vi "Просмотр графиков.vi"() -> ()   [LabVIEW 2011]
panel:
  out "т1 2":waveform(dbl)[](graph)
  out "т1":waveform(dbl)[](graph)
  in  "Закрыть окно":bool
  in  "Сохранить":bool
  # "С1"
  # "С2"
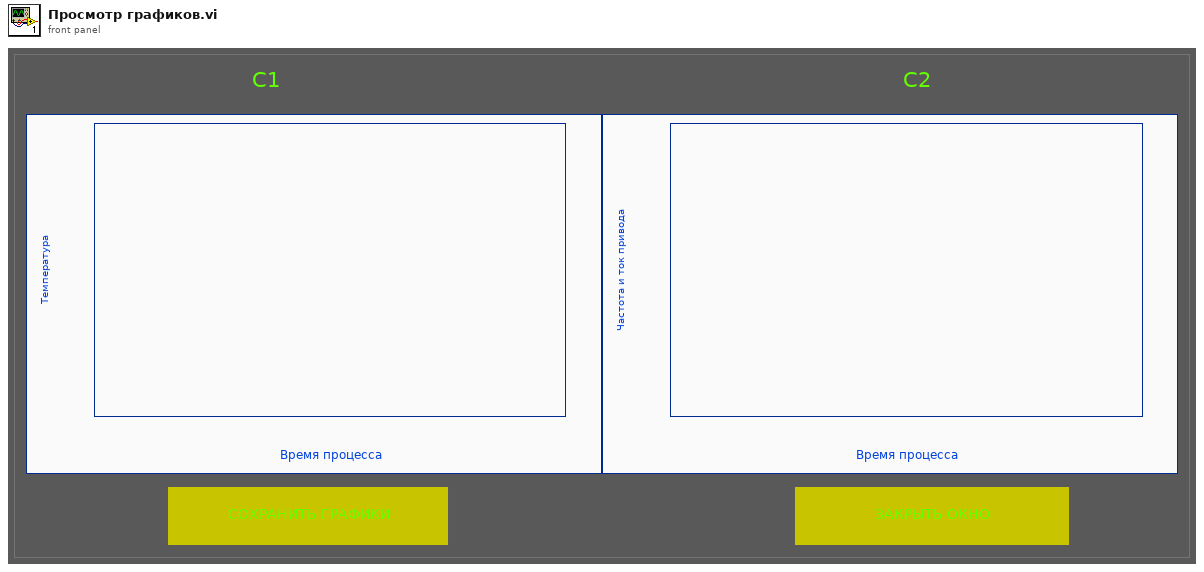
[diagram p1: front panel]
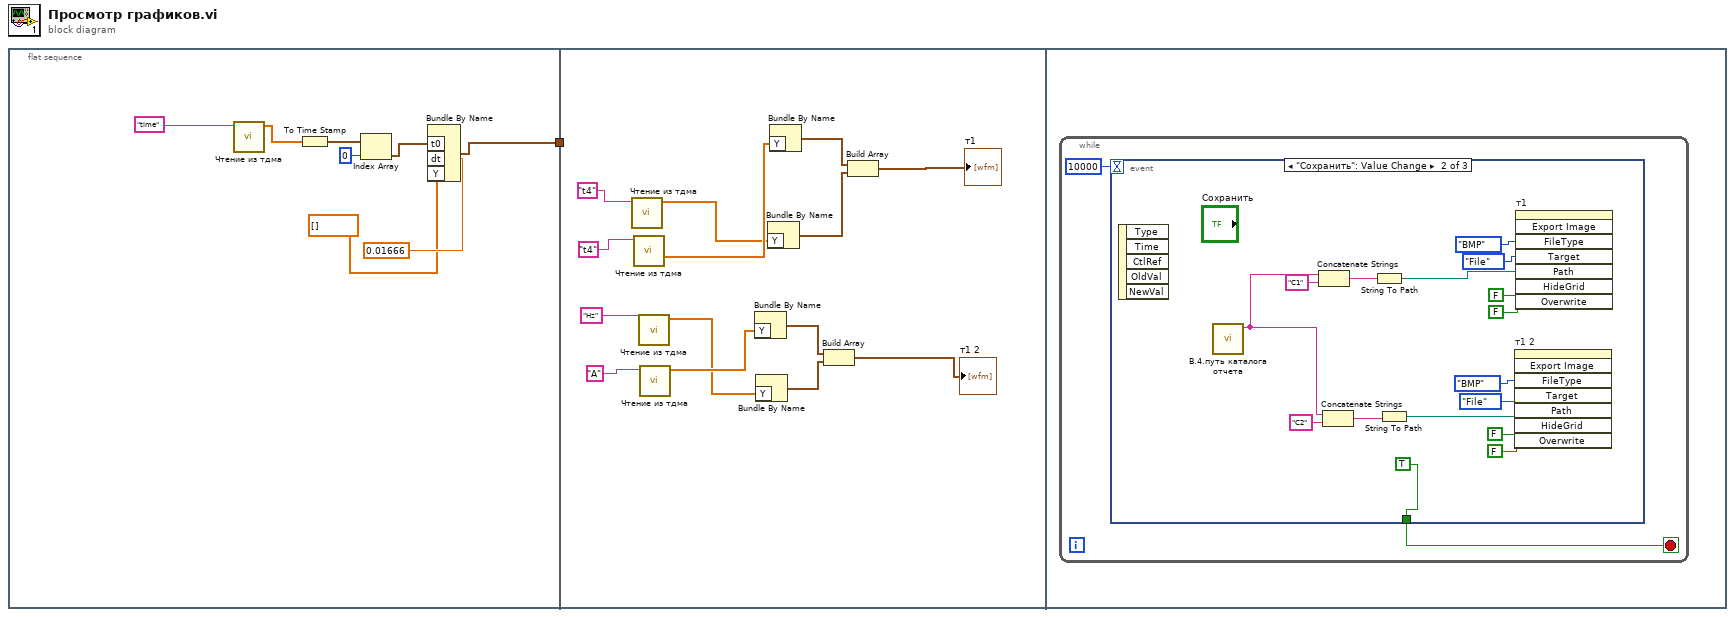
[diagram p0: block diagram]
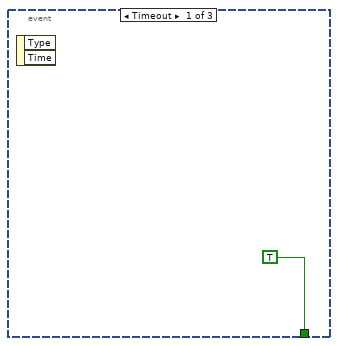
[diagram p2: hidden frame]
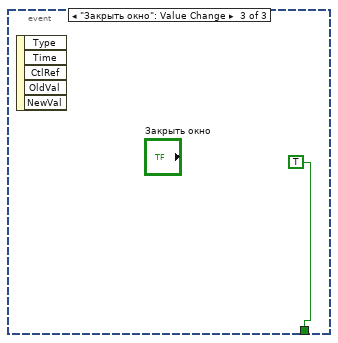
[diagram p3: hidden frame]
diagram:
  n1 = flat-sequence {
    tunnel: [w2] -> w1
    tunnel: w1 -> [_]
    frame #0 {
      n2 = call "Чтение из тдма.vi"("Канал"="time") -> ("data"=w7:dbl[])  [unwired: 10 in]
      n3 = To Time Stamp(1:w7) -> (0:w6:timestamp[])
      n4 = Index Array(array=w6, index=0) -> (element=w3:timestamp)
      n5 = Bundle By Name("t0"=w3, "dt"=0.01666, "Y"=dbl[] []) -> (w2:waveform(dbl))  [unwired: 1 in]
    }
    frame #1 {
      n6 = call "Чтение из тдма.vi"("Канал"="t4") -> ("data"=w10:dbl[])  [unwired: 10 in]
      n7 = call "Чтение из тдма.vi"("Канал"="t4") -> ("data"=w11:dbl[])  [unwired: 10 in]
      n8 = call "Чтение из тдма.vi"("Канал"="Hz") -> ("data"=w12:dbl[])  [unwired: 10 in]
      n9 = call "Чтение из тдма.vi"("Канал"="A") -> ("data"=w13:dbl[])  [unwired: 10 in]
      n10 = Bundle By Name("Y"=w13) -> (w15:waveform(dbl))  [unwired: 1 in]
      n11 = Bundle By Name("Y"=w12) -> (w16:waveform(dbl))  [unwired: 1 in]
      n12 = Bundle By Name("Y"=w10) -> (w20:waveform(dbl))  [unwired: 1 in]
      n13 = Bundle By Name("Y"=w11) -> (w21:waveform(dbl))  [unwired: 1 in]
      n14 = Build Array(w15, w16) -> (→"т1 2":waveform(dbl)[])
      n15 = Build Array(w21, w20) -> (→"т1":waveform(dbl)[])
    }
    frame #2 {
      n16 = while {
        stop <- w24 stop-if-true
        n17 = event shown="[1] \"Сохранить\": Value Change" {
          selector: _ -> [_ _ _]
          dyn-events: _ -> [_ _ _]
          timeout: 10000 -> [_ _ _]
          tunnel: [TRUE TRUE TRUE] -> w24
          event Timeout {
            n18 = event-data() -> ()  [unwired: 1 in, 2 out]
          }
          event "Сохранить": Value Change {
            n19 = event-data() -> ()  [unwired: 1 in, 5 out]
            n20 = call "B.4.путь каталога отчета.vi"() -> ("path_out"=w30:string)  [unwired: 11 in]
            n21 = Concatenate Strings(w30, "C1" ("string")) -> (w32:string)
            n22 = Concatenate Strings(w30, "C2" ("string")) -> (w34:string)
            n23 = String To Path(string=w32) -> (path=w31:path)
            n24 = String To Path(string=w34) -> (path=w33:path)
            n25 = invoke on="т1 2" class="WFGraph (strict)" method="Export Image"("FileType"=enum32{"BMP", "EPS", "EMF", "PICT"}."BMP" ("File Type"), "Target"=enum32{"File", "Clipboard"}."File", "Path"=w33, "HideGrid"=FALSE ("Hide Grid"), "Overwrite"=FALSE ("Always Overwrite")) -> ()  [unwired: 3 in, 8 out]
            n26 = invoke on="т1" class="WFGraph (strict)" method="Export Image"("FileType"=enum32{"BMP", "EPS", "EMF", "PICT"}."BMP" ("File Type"), "Target"=enum32{"File", "Clipboard"}."File", "Path"=w31, "HideGrid"=FALSE ("Hide Grid"), "Overwrite"=FALSE ("Always Overwrite")) -> ()  [unwired: 3 in, 8 out]
          }
          event "Закрыть окно": Value Change {
            n27 = event-data() -> ()  [unwired: 1 in, 5 out]
          }
        }
      }
    }
  }
